vi "WT-Controller-OL-NoDrag.vi"() -> ()   [LabVIEW 2016]
uses:
  <vilib>/Platform/TimedLoop/XDataNode/timing_clust.ctl
  <vilib>/Platform/TimedLoop/XDataNode/nitl_modes.ctl
  <vilib>/Platform/TimedLoop/XDataNode/wakeup.ctl
  <vilib>/platform/TimedLoop/XDataNode/XDataNode.xnode
  <vilib>/Platform/TimedLoop/XDataNode/XDNodeRunTimeDep.lvlib
panel:
  out "Velocity (mph)":dbl format="%0.2f"
  out "Boolean":bool
  in  "POWER":bool
  in  "Velocity (m/s)":dbl
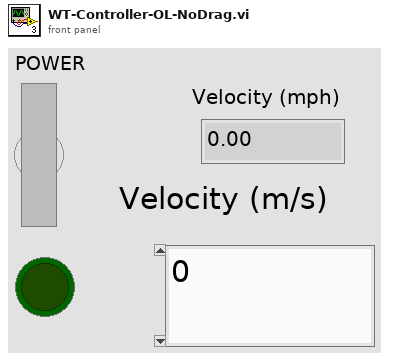
[diagram p1: front panel]
types:
  T1 = typedef "XDNodeRunTimeDep.lvlib/timing_clust.ctl" = cluster{"Expected End [f-1]":u64, "Actual End [f-1]":u64, "Finished Late? [f-1]":bool, "Expected End [i-1]":u64, "Actual End [i-1]":u64, "Finished Late? [i-1]":bool, "Expected Start [i]":u64, "Actual Start [i]":u64, "Expected Start [f]":u64, "Actual Start [f]":u64, "Source Name":string, "Structure Name":string, "Period":i64, "Deadline":i64, "Offset":i64, "Start":i64, "Priority":i32, "Timeout":i32, "Mode":T2, "Wakeup Reason":T3, "Error":errorcluster, "Source Type":string, "Secondary Source Type":string, "Global End Time":u64, "Global Start Time":u64, "Frame Duration":u64, "Iteration Duration":u64, "Assigned CPU":i32, "I/O Scan Engine Mode":u32}
  T2 = typedef "XDNodeRunTimeDep.lvlib/nitl_modes.ctl" = enum32{"No Change", "Process missed periods, maintain original phase", "Discard missed periods, maintain original phase", "Process missed periods, ignore original phase", "Discard missed periods, ignore original phase"}
  T3 = typedef "XDNodeRunTimeDep.lvlib/wakeup.ctl" = enum32{"Normal", "Aborted", "Asynchronous wakeup", "Timing source error", "Timed loop error", "Timeout"}
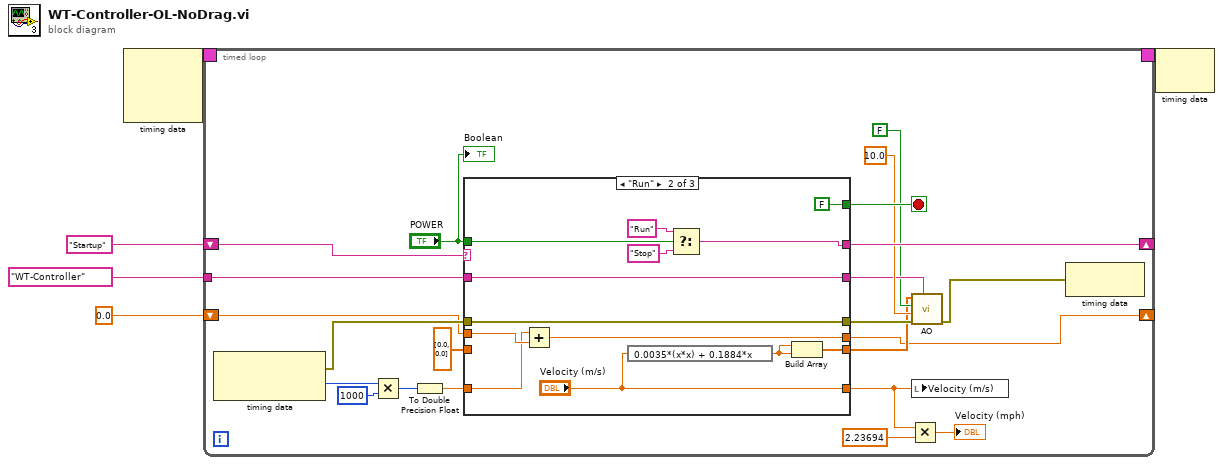
[diagram p0: block diagram]
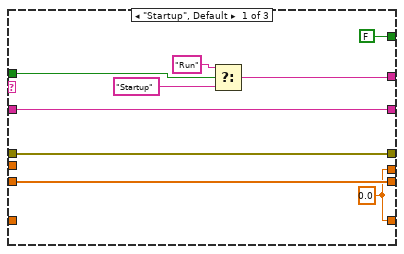
[diagram p2: hidden frame]
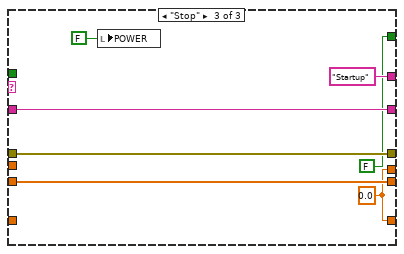
[diagram p3: hidden frame]
diagram:
  n1 = node-c288() -> (w3:T1)  [unwired: 3 in]
  n2 = timed-loop {
    shift-right: [w26] -> _
    shift-left: "Startup" -> [w27]
    tunnel: tag "WT-Controller" ("device name") -> [w24]
    timing: w3 -> [_]
    timing-out: [_] -> w2
    shift-right: [w10] -> _
    shift-left: 0.0 -> [w12]
    stop <- w25 stop-if-true
    n3 = node-c288() -> (w19:errorcluster, w15:i64)  [unwired: 1 in]
    n4 = Multiply(x=w15, y=i64 1000) -> (x*y=w13:i64)
    n5 = To Double Precision Float(number=w13) -> (double precision float=w11:dbl)
    n6 = case shown="\"Run\"" w27 {
      tunnel: [w36 w55 "Startup" ("f")] -> w26
      tunnel: [w41 w53 w60] -> w16
      tunnel: [FALSE ("Stop") FALSE ("Stop") FALSE ("Stop")] -> w25
      tunnel: w24 -> [w40 w52 w61]
      tunnel: [w42 w51 w59] -> w21
      tunnel: w19 -> [w42 w51 w59]
      tunnel: dbl[] [0.0, 0.0] ("appended array") -> [w41 _ w60]
      tunnel: [w40 w52 w61] -> w20
      tunnel: "POWER" -> [w38 w50 _]
      tunnel: w12 -> [_ w47 _]
      tunnel: [w34 w45 w56] -> w10
      tunnel: w11 -> [_ w46 _]
      tunnel: [w34 "Velocity (m/s)" w56] -> w9
      frame "Startup", Default {
        w34 = 0.0
        n7 = Select(t="Run" ("f"), s=w38, f="Startup") -> (s? t:f=w36:string)
      }
      frame "Run" {
        n8 = Add(x=w46, y=w47) -> (x+y=w45:dbl)
        n9 = expression code="0.0035*(x*x) + 0.1884*x"("Velocity (m/s)") -> (w44:dbl)
        n10 = Select(t="Run" ("f"), s=w50, f="Stop") -> (s? t:f=w55:string)
        n11 = Build Array(w44, w44) -> (w53:dbl[])
      }
      frame "Stop" {
        w56 = 0.0
        n12 = local write "POWER"(FALSE ("POWER")) -> ()
      }
    }
    n13 = Multiply(x=w9, y=2.23694) -> (x*y=→"Velocity (mph)":dbl)
    n14 = call "AO.vi"("device name"=w20, "error in"=w21, "timeout (s)"=10.0, "stop (T)"=FALSE, "data"=w16) -> ("error out"=w6:errorcluster)  [unwired: 2 in, 1 out]
    n15 = local write "Velocity (m/s)"(w9) -> ()
    n16 = node-c288(w6) -> ()  [unwired: 1 out]
    "Boolean" <- "POWER"
  }
  n17 = node-c288(w2) -> ()  [unwired: 1 out]
